vi "RT Driver VI.vi"(6 "Device Clock":string, 9 "Device Inputs FIFO":refnum<k33>, 10 "Device Outputs FIFO":refnum<k33>, 11 "Device Reference":T1 format="%.0x") -> ()   [LabVIEW 2019, in "RefMem DMA Engine.lvlib"]
uses:
  RefMem DMA Engine.lvlib
  <vilib>/NI VeriStand/Custom Device API/Custom Device Item Ref.ctl
  <vilib>/NI VeriStand/Custom Device API/Custom Device Channel Type.ctl
  <vilib>/Platform/TimedLoop/XDataNode/timing_clust.ctl
  <vilib>/Platform/TimedLoop/XDataNode/nitl_modes.ctl
  <vilib>/Platform/TimedLoop/XDataNode/wakeup.ctl
  5565/GE5565 Set DMA Transfer Size.vi
  5565/GE5565 Write (U64) Cluster.vi
  SubVIs/Decimation - time to write.vi
  5565/GE5565 Set DMA RW (Cluster) mod.vi
  5565/GE5565 DMA Read Interrupt (U64) Cluster.vi
  Shared/Constants.vi
  <vilib>/NI VeriStand/Custom Device Tools/Custom Device Utility Library/NI VeriStand - Search for Item.vi
  <vilib>/NI VeriStand/Custom Device Tools/Custom Device Utility Library/NI VeriStand - Search for Item by Name.vi
  <vilib>/NI VeriStand/Custom Device Tools/Custom Device Utility Library/NI VeriStand - Get Channel FIFO Buffer Index.vi
  <vilib>/NI VeriStand/Custom Device API/Get Item Property (I32).vi
  <vilib>/NI VeriStand/Custom Device API/Get Item Property (String).vi
  <vilib>/Platform/TimedLoop/XDataNode/XDataNode.xnode
  <vilib>/Platform/TimedLoop/XDataNode/XDNodeRunTimeDep.lvlib
  <vilib>/NI VeriStand/Custom Device API/Custom Device API.lvlib
  <vilib>/NI VeriStand/Custom Device Tools/Custom Device Utility Library/Custom Device Utility Library.lvlib
  Shared/RefMem DMA Shared.lvlib
  Shared/Block descriptor.ctl
  <vilib>/Platform/TimedLoop/scheduler/LVUserAPI/_suppVIs/Create_1MHz_TSource.vi
panel:
  out "Write Duration (us)":u32
  in  "stop":bool
  out "error out":errorcluster
  in  "Status Notifier":refnum<notifier>
  # "Use this template as a starting point for creating a custom device code module. The input controls shown here are specially named controls that the system will use to provide the device loop with data. The controls are not required for the device loop to run. For instance, if the device doesn't produce any output data, then you don't need the Device Outputs FIFO control. If you do use these controls, however, they need to have these exact names to be functional."
  # "The optional status notifier element is used to notify the RT engine of the last state of the custom device, and to indicate the device has completed execution. If this control is not used, a default No Error value is returned to the system when the device finishes execution.\n\nNote: This error state is not checked until the system shuts down. Use an output status channel to send more immediate status values to the system."
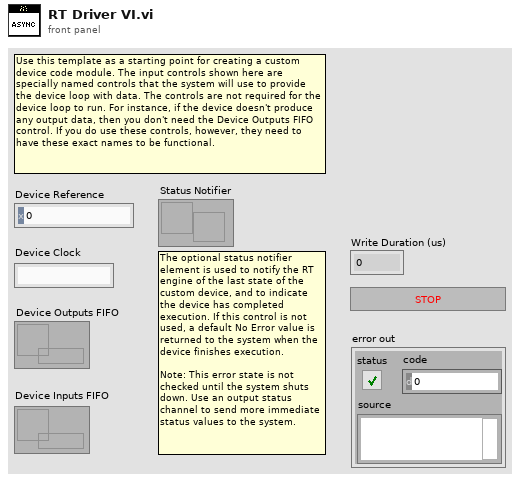
[diagram p1: front panel]
types:
  T1 = typedef "Custom Device API.lvlib/Custom Device Item Ref.ctl" = u64
  T2 = typedef "Custom Device API.lvlib/Custom Device Channel Type.ctl" = enum16{"Input", "Output"}
  T3 = enum16{"open", "replace", "create", "open or create", "replace or create", "replace or create with confirmation"}
  T4 = typedef "RefMem DMA Shared.lvlib/Block descriptor.ctl" = cluster{"Block Address in Bytes":u32, "Block Decimation \nchannel index":i32, "Transfer size":u32, "FIFO Indexes":i32[], "Channel index in block":i32[]}
  T5 = cluster{"VMIC 5565 Resource":refnum<visa-resource-name>, "MEMACC Resource":refnum<visa-resource-name>, "byte count":u32, "mem offset":u32}
  T6 = typedef "Custom Device API.lvlib/Custom Device Timed Loop Priority.ctl" = enum32{"Low", "Medium", "High"}
  T7 = typedef "XDNodeRunTimeDep.lvlib/timing_clust.ctl" = cluster{"Expected End [f-1]":u64, "Actual End [f-1]":u64, "Finished Late? [f-1]":bool, "Expected End [i-1]":u64, "Actual End [i-1]":u64, "Finished Late? [i-1]":bool, "Expected Start [i]":u64, "Actual Start [i]":u64, "Expected Start [f]":u64, "Actual Start [f]":u64, "Source Name":string, "Structure Name":string, "Period":i64, "Deadline":i64, "Offset":i64, "Start":i64, "Priority":i32, "Timeout":i32, "Mode":T8, "Wakeup Reason":T9, "Error":errorcluster, "Source Type":string, "Secondary Source Type":string, "Global End Time":u64, "Global Start Time":u64, "Frame Duration":u64, "Iteration Duration":u64, "Assigned CPU":i32, "I/O Scan Engine Mode":u32}
  T8 = typedef "XDNodeRunTimeDep.lvlib/nitl_modes.ctl" = enum32{"No Change", "Process missed periods, maintain original phase", "Discard missed periods, maintain original phase", "Process missed periods, ignore original phase", "Discard missed periods, ignore original phase"}
  T9 = typedef "XDNodeRunTimeDep.lvlib/wakeup.ctl" = enum32{"Normal", "Aborted", "Asynchronous wakeup", "Timing source error", "Timed loop error", "Timeout"}
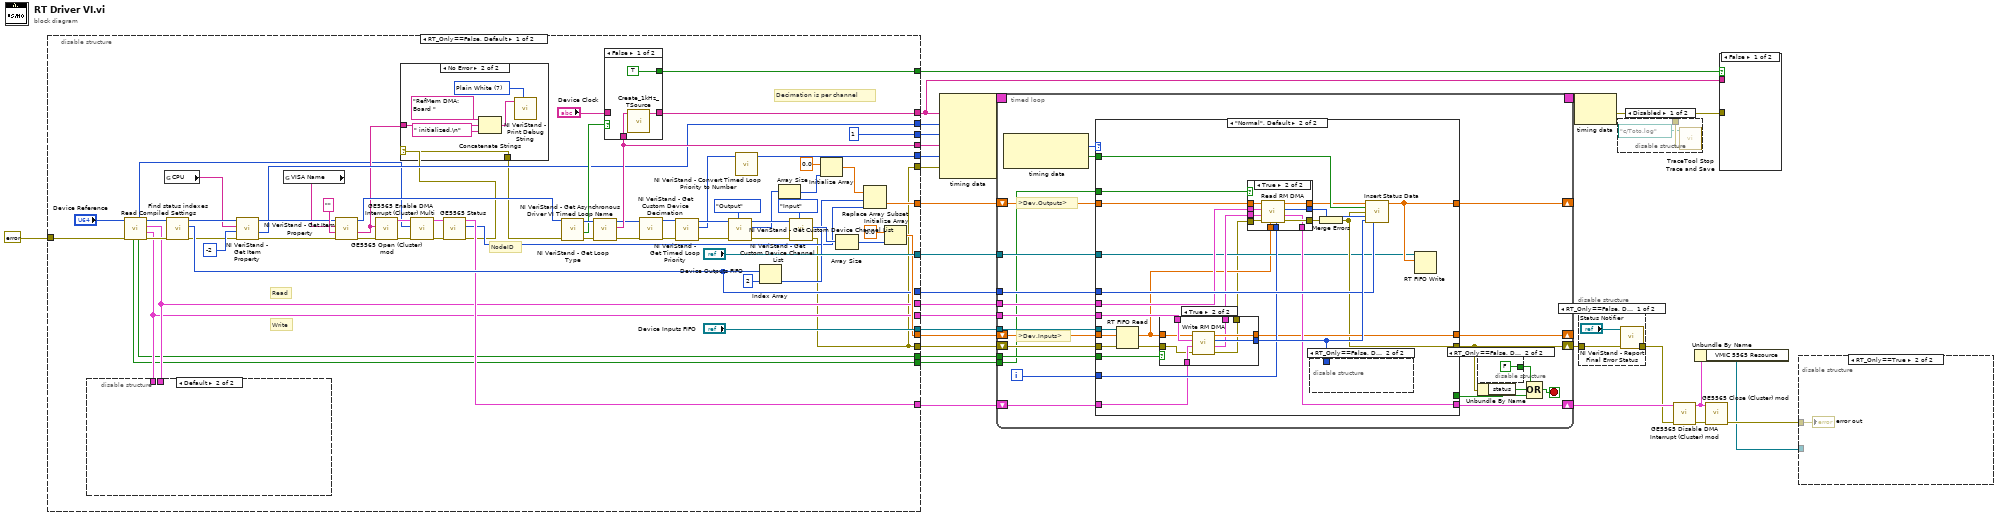
[diagram p0: block diagram]
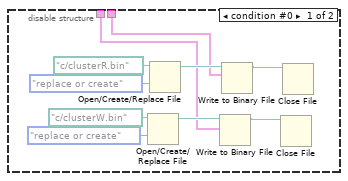
[diagram p3: hidden frame]
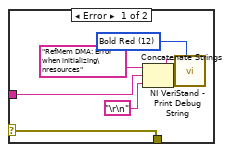
[diagram p4: hidden frame]
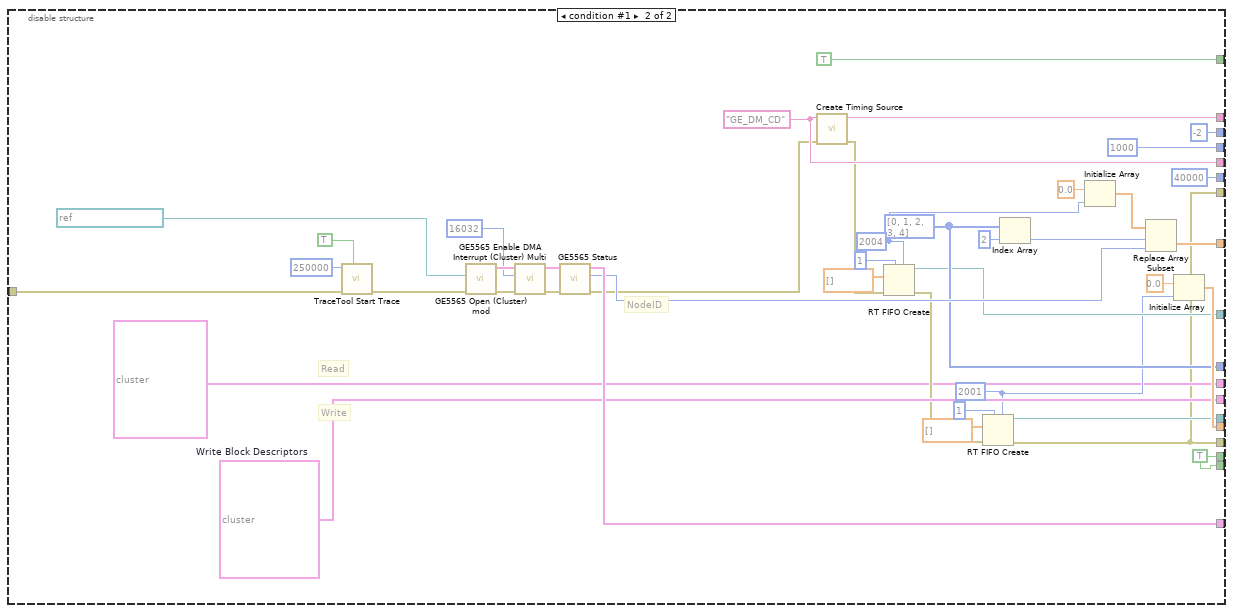
[diagram p6: hidden frame]
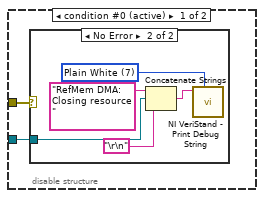
[diagram p7: hidden frame]
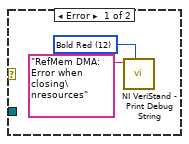
[diagram p8: hidden frame]
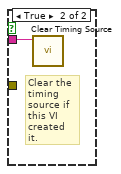
[diagram p10: hidden frame]
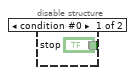
[diagram p11: hidden frame]
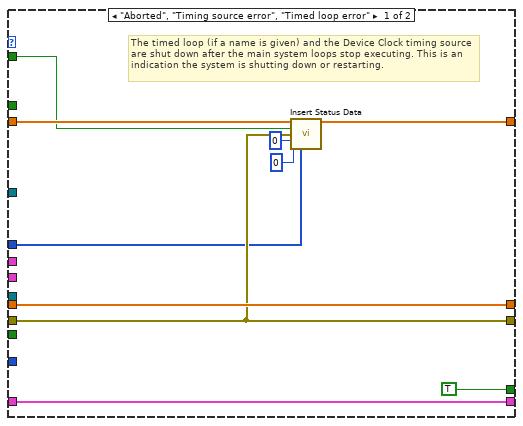
[diagram p12: hidden frame]
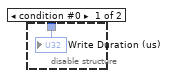
[diagram p13: hidden frame]
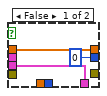
[diagram p14: hidden frame]
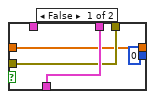
[diagram p15: hidden frame]
diagram:
  n1 = disable-structure shown="RT_Only==False, Default" {
    disable-tunnel: ["Device Outputs FIFO" w131] -> w29
    disable-tunnel: ["Device Inputs FIFO" w128] -> w28
    disable-tunnel: [w89 w158] -> w25
    disable-tunnel: [w80 40000 ("Numeric Priority")] -> w24
    disable-tunnel: [w74 TRUE] -> w23
    disable-tunnel: [w73 w156] -> w22
    disable-tunnel: [w72 w144] -> w21
    disable-tunnel: [w64 w154] -> w20
    disable-tunnel: [w59 w140] -> w19
    disable-tunnel: [w55 -2 ("Value")] -> w18
    disable-tunnel: [i64 1 ("Period") i64 1000 ("Period")] -> w17
    disable-tunnel: [w49 w146] -> w16
    disable-tunnel: [w30 w124] -> w8
    disable-tunnel: [w36 T4[] [{"Block Address in Bytes"=0, "Block Decimation \nchannel index"=2001, "Transfer size"=16000, "FIFO Indexes"=array[2000 elements], "Channel index in block"=array[2000 elements]}] ("Read Block Descriptors")] -> w7
    disable-tunnel: [w35 w139] -> w6
    disable-tunnel: [w34 w143] -> w5
    disable-tunnel: [w33 w143] -> w4
    disable-tunnel: errorcluster {"status"=FALSE, "code"=0, "source"=""} ("error in (no error)") -> [w31 w123]
    disable-tunnel: [w30 w124] -> w2
    frame condition #0 (active) {
      # "Write"
      # "Read"
      # "Decimation is per channel"
      # "NodeID"
      n2 = call "Read Compiled Settings.vi"("error in (no error)"=w31, "Device Reference In"="Device Reference") -> ("error out"=w39:errorcluster, "Write Block Descriptors"=w35:T4[], "Read Block Descriptors"=w36:T4[], "Device Reference Out"=w37:T1, "Write"=w33:bool, "max channel count bytes"=w32:u32, "Read"=w34:bool)  [unwired: 3 in]
      n3 = disable-structure shown="Default" {
        disable-tunnel: w36 -> [w99 _]
        disable-tunnel: w35 -> [w94 _]
        frame condition #0 {
          n4 = Open/Create/Replace File(file path (use dialog)=path "c:/clusterW.bin", operation (0:open)=T3."replace or create") -> (refnum out=w95:refnum<file>)  [unwired: 4 in, 2 out]
          n5 = Open/Create/Replace File(file path (use dialog)=path "c:/clusterR.bin", operation (0:open)=T3."replace or create") -> (refnum out=w103:refnum<file>)  [unwired: 4 in, 2 out]
          n6 = Write to Binary File(file (use dialog)=w95, data=w94) -> (refnum out=w98:refnum<file>)  [unwired: 4 in, 2 out]
          n7 = Write to Binary File(file (use dialog)=w103, data=w99) -> (refnum out=w100:refnum<file>)  [unwired: 4 in, 2 out]
          n8 = Close File(refnum=w98) -> ()  [unwired: 1 in, 2 out]
          n9 = Close File(refnum=w100) -> ()  [unwired: 1 in, 2 out]
        }
        frame condition #1 (active) {
        }
      }
      n10 = global read "Constants.vi" "CPU"() -> (w42:string)
      n11 = call "Find status indexes.vi"("error in (no error)"=w39, "Custom Device ref"=w37) -> ("error out"=w44:errorcluster, "Indexes"=w59:i32[], "Custom Device ref"=w58:T1)  [unwired: 7 in]
      n12 = call-poly <vilib>:"NI VeriStand - Get Item Property.vi"("error in (no error)"=w44, "Default Value"=-2 ("Automatic Processor"), "Property Name"=w42, "Item Ref in"=w58) -> ("error out"=w43:errorcluster, "Value"=w55:i32, "Item Ref out"=w56:T1)  [unwired: 4 in, 1 out]
      n13 = global read "Constants.vi" "VISA Name"() -> (w40:string)
      n14 = call-poly <vilib>:"NI VeriStand - Get Item Property.vi"("error in (no error)"=w43, "Default Value"="", "Property Name"=w40, "Item Ref in"=w56) -> ("error out"=w48:errorcluster, "Value"=w41:string, "Item Ref out"=w66:T1)  [unwired: 4 in, 1 out]
      n15 = call "GE5565 Open (Cluster) mod.vi"("error in (no error)"=w48, "VISA resource name (empty)"=w41) -> ("error out"=w53:errorcluster, "VMIC-5565"=w52:T5)  [unwired: 4 in]
      n16 = call "GE5565 Enable DMA Interrupt (Cluster) Multi.vi"("error in (no error)"=w53, "transfer size (1024 bytes)"=w32, "VMIC reference in"=w52) -> ("error out"=w51:errorcluster, "VMIC reference out"=w50:T5)  [unwired: 3 in]
      n17 = call "GE5565 Status.vi"("error in (no error)"=w51, "VMIC reference in"=w50) -> ("error out"=w46:errorcluster, "Node ID"=w47:u8, "VMIC reference out"=w49:T5)  [unwired: 3 in]
      n18 = case shown="No Error" w46 {
        selector: w46 -> [w108 w114]
        tunnel: [w108 w114] -> w45
        tunnel: w41 -> [w105 w110]
        frame Error {
          w109 = u16 12 items=["Plain White"=7, "Bold White"=15, "Bold Blue"=9, "Bold Green"=10, "Bold Red"=12] ("Color (Plain White)")
          n19 = Concatenate Strings("RefMem DMA: Error when initializing\nresources" ("Debug String"), w105, "\r\n") -> (w107:string)
          n20 = call <vilib>:"NI VeriStand - Print Debug String.vi"("Attribute"=w109, "Message"=w107) -> ()  [unwired: 9 in, 1 out]
        }
        frame No Error {
          w115 = u16 7 items=["Plain White"=7, "Bold White"=15, "Bold Blue"=9, "Bold Green"=10, "Bold Red"=12] ("Color (Plain White)")
          n21 = Concatenate Strings("RefMem DMA: Board " ("Debug String"), w110, " initialized.\n" ("string")) -> (w112:string)
          n22 = call <vilib>:"NI VeriStand - Print Debug String.vi"("Attribute"=w115, "Message"=w112) -> ()  [unwired: 9 in, 1 out]
        }
      }
      n23 = call <vilib>:"NI VeriStand - Get Loop Type.vi"("error in (no error)"=w45, "Device Ref in"=w66) -> ("error out"=w78:errorcluster, "Use Device Clock"=w76:bool, "Device Ref out"=w77:T1)  [unwired: 7 out]
      n24 = call <vilib>:"NI VeriStand - Get Asynchronous Driver VI Timed Loop Name.vi"("error in (no error)"=w78, "Device Ref in"=w77) -> ("error out"=w71:errorcluster, "Device Timed Loop Name"=w72:string, "Device Ref out"=w70:T1)  [unwired: 7 out]
      n25 = case shown="False" w76 {
        tunnel: "Device Clock" -> [_ w119]
        tunnel: [w118 w119] -> w73
        tunnel: [TRUE _] -> w74
        tunnel: w72 -> [w116 _]
        frame False {
          n26 = call <vilib>:"Create_1kHz_TSource.vi"("name (in)"=w116) -> ("name (out)"=w118:string)  [unwired: 1 in, 9 out]
        }
        frame True {
        }
      }
      n27 = call <vilib>:"NI VeriStand - Get Custom Device Decimation.vi"("error in (no error)"=w71, "Device Ref in"=w70) -> ("error out"=w68:errorcluster, "Device Ref out"=w69:T1)  [unwired: 7 in, 1 out]
      n28 = call <vilib>:"NI VeriStand - Get Timed Loop Priority.vi"("error in (no error)"=w68, "Device Ref in"=w69) -> ("error out"=w83:errorcluster, "Priority"=w81:T6, "Device Ref out"=w84:T1)  [unwired: 7 out]
      n29 = call <vilib>:"NI VeriStand - Get Custom Device Channel List.vi"("Channel Type"=Custom_Device_Channel_Type."Output", "error in (no error)"=w83, "Device Ref in"=w84) -> ("error out"=w86:errorcluster, "Specified Channel Ref List"=w60:T1[], "Device Ref out"=w87:T1)  [unwired: 6 out]
      n30 = call <vilib>:"NI VeriStand - Convert Timed Loop Priority to Number.vi"("Priority"=w81) -> ("Numeric Priority"=w80:i32)  [unwired: 10 out]
      n31 = Index Array(array=w59, index=2) -> (element=w61:i32)
      n32 = Array Size(array=w60) -> (size(s)=w63:i32)
      n33 = call <vilib>:"NI VeriStand - Get Custom Device Channel List.vi"("Channel Type"=Custom_Device_Channel_Type."Input", "error in (no error)"=w86, "Device Ref in"=w87) -> ("error out"=w30:errorcluster, "Specified Channel Ref List"=w82:T1[])  [unwired: 7 out]
      n34 = Initialize Array(0.0 ("element"), w63) -> (w65:dbl[])
      n35 = Array Size(array=w82) -> (size(s)=w79:i32)
      n36 = Replace Array Subset(array=w65, new element=w47, index=w61) -> (w64:dbl[])
      n37 = Initialize Array(0.0 ("element"), w79) -> (w89:dbl[])
    }
    frame condition #1 {
      w139 = T4[] [{"Block Address in Bytes"=0, "Block Decimation \nchannel index"=0, "Transfer size"=16000, "FIFO Indexes"=array[2000 elements], "Channel index in block"=array[2000 elements]}]  # Write Block Descriptors
      w126 = u32 2001 ("elements in array (1)")
      w132 = u32 2004 ("elements in array (1)")
      w140 = i32[] [0, 1, 2, 3, 4]
      w143 = TRUE ("Write")
      w144 = "GE_DM_CD" ("Device Timed Loop Name")
      # "Write"
      # "Read"
      # "NodeID"
      n38 = call <vilib>:"TraceTool Start Trace.vi"("Detailed Tracing? (F)"=TRUE, "error in (no error)"=w123, "Buffer Size (250000 bytes)"=250000) -> ("error out"=w122:errorcluster)  [unwired: 7 in, 1 out]
      n39 = call "GE5565 Open (Cluster) mod.vi"("error in (no error)"=w122, "VISA resource name (empty)"=refnum<visa-resource-name> "PXI2::15::INSTR") -> ("error out"=w150:errorcluster, "VMIC-5565"=w149:T5)  [unwired: 4 in]
      n40 = call "GE5565 Enable DMA Interrupt (Cluster) Multi.vi"("error in (no error)"=w150, "transfer size (1024 bytes)"=u32 16032, "VMIC reference in"=w149) -> ("error out"=w148:errorcluster, "VMIC reference out"=w147:T5)  [unwired: 3 in]
      n41 = call "GE5565 Status.vi"("error in (no error)"=w148, "VMIC reference in"=w147) -> ("error out"=w137:errorcluster, "Node ID"=w145:u8, "VMIC reference out"=w146:T5)  [unwired: 3 in]
      n42 = call-poly <vilib>:"Create Timing Source.vi"("error in (no error)"=w137, "name (in)"=w144) -> ("error out"=w135:errorcluster, "name (out)"=w156:string)  [unwired: 8 in]
      n43 = RT FIFO Create(1:dbl[] [], 3:w135, 4:u32 1 ("size (10)"), 6:w132) -> (8:w131:refnum<k33>, 11:w127:errorcluster)  [unwired: 4 in, 1 out]
      n44 = RT FIFO Create(1:dbl[] [], 3:w127, 4:u32 1 ("size (10)"), 6:w126) -> (8:w128:refnum<k33>, 11:w124:errorcluster)  [unwired: 4 in, 1 out]
      n45 = Index Array(array=w140, index=2) -> (element=w152:i32)
      n46 = Initialize Array(0.0 ("element"), w132) -> (w155:dbl[])
      n47 = Replace Array Subset(array=w155, new element=w145, index=w152) -> (w154:dbl[])
      n48 = Initialize Array(0.0 ("element"), w126) -> (w158:dbl[])
    }
  }
  n49 = node-c288(w22, w18, w17, w21, w24, w2) -> (w27:T7)
  n50 = timed-loop {
    timing: w27 -> [_]
    timing-out: [_] -> w26
    shift-right: [w180] -> _
    shift-left: w25 -> [w181]
    shift-right: [w177] -> _
    shift-left: w20 -> [w178]
    tunnel: w29 -> [w176]
    tunnel: w28 -> [w175]
    tunnel: w19 -> [w169]
    shift-right: [w166] -> w14
    shift-left: w16 -> [w168]
    shift-right: [w174] -> w11
    shift-left: w8 -> [w182]
    tunnel: w6 -> [w165]
    tunnel: w7 -> [w164]
    tunnel: w4 -> [w163]
    tunnel: w5 -> [w162]
    i -> [w167]
    stop <- w171 stop-if-true
    # ">Dev.Outputs>"
    # ">Dev.Inputs>"
    n51 = node-c288() -> (w179:T9, w170:bool)  [unwired: 1 out]
    n52 = case shown="\"Normal\", Default" w179 {
      tunnel: w182 -> [w188 w198]
      tunnel: w181 -> [w194 w199]
      tunnel: [w188 w202] -> w174
      tunnel: [w194 w203] -> w180
      tunnel: w178 -> [w191 w219]
      tunnel: [w190 w218] -> w177
      tunnel: w176 -> [_ w201]
      tunnel: w175 -> [_ w200]
      tunnel: [TRUE _] -> w172
      tunnel: w170 -> [w189 w216]
      tunnel: w169 -> [w185 w213]
      tunnel: w168 -> [w192 w210]
      tunnel: w167 -> [_ w211]
      tunnel: [w192 w208] -> w166
      tunnel: w165 -> [_ w207]
      tunnel: w164 -> [_ w206]
      tunnel: w163 -> [_ w205]
      tunnel: w162 -> [_ w204]
      frame "Aborted", "Timing source error", "Timed loop error" {
        # "The timed loop (if a name is given) and the Device Clock timing source are shut down after the main system loops stop executing. This is an indication the system is shutting down or restarting."
        n53 = call "Insert Status Data.vi"("OutputData in"=w191, "Late?"=w189, "error in (no error)"=w188, "Read Duration"=u32 0, "Write Duration"=u32 0, "Status Channel Indexes"=w185) -> ("OutputData out"=w190:dbl[])  [unwired: 9 in]
      }
      frame "Normal", Default {
        n54 = RT FIFO Read(0:w200, 1:w199, 3:w198) -> (9:w196:dbl[], 11:w197:errorcluster)  [unwired: 4 out]
        n55 = case shown="True" w205 {
          tunnel: w196 -> [w235 w239]
          tunnel: w197 -> [w236 w238]
          tunnel: [w235 w245] -> w203
          tunnel: [u32 0 ("Write Duration") w244] -> w217
          tunnel: [w236 w243] -> w195
          tunnel: w210 -> [w237 w242]
          tunnel: [w237 w241] -> w209
          tunnel: w207 -> [_ w240]
          frame False {
          }
          frame True {
            n56 = call "Write RM DMA.vi"("error in"=w238, "VMIC reference in"=w242, "Block descriptors"=w240, "Values"=w239) -> ("error out"=w243:errorcluster, "VMIC reference out"=w241:T5, "Write Duration"=w244:u32, "Values"=w245:dbl[])  [unwired: 4 in]
          }
        }
        n57 = case shown="True" w204 {
          tunnel: w219 -> [w223 w233]
          tunnel: [w223 w232] -> w215
          tunnel: [u32 0 ("Read Duration") w231] -> w214
          tunnel: [_ w230] -> w212
          tunnel: w211 -> [_ w229]
          tunnel: w209 -> [w221 w228]
          tunnel: [w221 w227] -> w208
          tunnel: w206 -> [_ w226]
          tunnel: w196 -> [_ w225]
          tunnel: w195 -> [_ w224]
          frame False {
          }
          frame True {
            n58 = call "Read RM DMA.vi"("Iteration"=w229, "Read Values"=w225, "error in"=w224, "VMIC reference in"=w228, "Block descriptors"=w226, "Old Values"=w233) -> ("error out"=w230:errorcluster, "VMIC reference out"=w227:T5, "Read Duration"=w231:u32, "Updated Values"=w232:dbl[])  [unwired: 2 in]
          }
        }
        n59 = disable-structure shown="RT_Only==False, Default" {
          disable-tunnel: w217 -> [w220 _]
          frame condition #0 {
            "Write Duration (us)" <- w220
          }
          frame condition #1 (active) {
          }
        }
        n60 = Merge Errors(w212) -> (w202:errorcluster)
        n61 = call "Insert Status Data.vi"("OutputData in"=w215, "Late?"=w216, "error in (no error)"=w202, "Read Duration"=w214, "Write Duration"=w217, "Status Channel Indexes"=w213) -> ("OutputData out"=w218:dbl[])  [unwired: 9 in]
        n62 = RT FIFO Write(0:w201, 1:w218) -> ()  [unwired: 2 in, 5 out]
      }
    }
    n63 = Unbundle By Name(w174) -> ("status"=w173:bool)
    n64 = disable-structure shown="RT_Only==False, Default" {
      disable-tunnel: ["stop" FALSE ("stop")] -> w161
      frame condition #0 {
      }
      frame condition #1 (active) {
      }
    }
    n65 = Compound Arithmetic op=OR(w161, w173, w172) -> (w171:bool)
  }
  n66 = node-c288(w26) -> (w1:errorcluster)
  n67 = disable-structure shown="RT_Only==False, Default" {
    disable-tunnel: [w251 w253] -> w13
    disable-tunnel: w11 -> [w250 w253]
    frame condition #0 (active) {
      n68 = call <vilib>:"NI VeriStand - Report Final Error Status.vi"("error in (no error)"=w250, "Status Notifier"="Status Notifier") -> ("error out"=w251:errorcluster)  [unwired: 1 in, 8 out]
    }
    frame condition #1 {
    }
  }
  n69 = disable-structure shown="Disabled" {
    disable-tunnel: w1 -> [w255 _]
    frame Disabled {
      n70 = call <vilib>:"TraceTool Stop Trace and Save.vi"("error in (no error)"=w255, "Path to Trace Log"=path "c:/Toto.log" ("Trace Host Network Address")) -> ()  [unwired: 9 in, 1 out]
    }
    frame Enabled {
    }
  }
  n71 = call "GE5565 Disable DMA Interrupt (Cluster) mod.vi"("error in (no error)"=w13, "VMIC reference in"=w14) -> ("error out"=w15:errorcluster, "VMIC reference out"=w10:T5)  [unwired: 4 in]
  n72 = Unbundle By Name(w10) -> ("VMIC 5565 Resource"=w9:refnum<visa-resource-name>)
  n73 = call "GE5565 Close (Cluster) mod.vi"("error in (no error)"=w15, "VMIC reference in"=w10) -> ("error out"=w12:errorcluster)  [unwired: 5 in]
  n74 = case shown="False" w23 {
    tunnel: w1 -> [_ _]
    tunnel: w22 -> [_ w256]
    frame False {
    }
    frame True {
      # "Clear the timing source if this VI created it."
      n75 = call <vilib>:"Clear Timing Source.vi"("name"=w256) -> ()  [unwired: 1 in, 10 out]
    }
  }
  n76 = disable-structure shown="RT_Only==True" {
    disable-tunnel: w12 -> [w258 w266]
    disable-tunnel: w9 -> [w257 _]
    frame condition #0 (active) {
      n77 = case shown="No Error" w258 {
        tunnel: w257 -> [_ w262]
        frame Error {
          w260 = u16 12 items=["Plain White"=7, "Bold White"=15, "Bold Blue"=9, "Bold Green"=10, "Bold Red"=12] ("Color (Plain White)")
          n78 = call <vilib>:"NI VeriStand - Print Debug String.vi"("Attribute"=w260, "Message"="RefMem DMA: Error when closing\nresources" ("Debug String")) -> ()  [unwired: 9 in, 1 out]
        }
        frame No Error {
          w265 = u16 7 items=["Plain White"=7, "Bold White"=15, "Bold Blue"=9, "Bold Green"=10, "Bold Red"=12] ("Color (Plain White)")
          n79 = Concatenate Strings("RefMem DMA: Closing resource " ("Debug String"), w262, "\r\n") -> (w263:string)
          n80 = call <vilib>:"NI VeriStand - Print Debug String.vi"("Attribute"=w265, "Message"=w263) -> ()  [unwired: 9 in, 1 out]
        }
      }
    }
    frame condition #1 {
      "error out" <- w266
    }
  }
